vi "Capture Image.vi"(8 "Error In":errorcluster) -> (0 "Error Out":errorcluster)   [LabVIEW 2014]
uses:
  <vilib>/httpClient/LabVIEWHTTPClient.lvlib
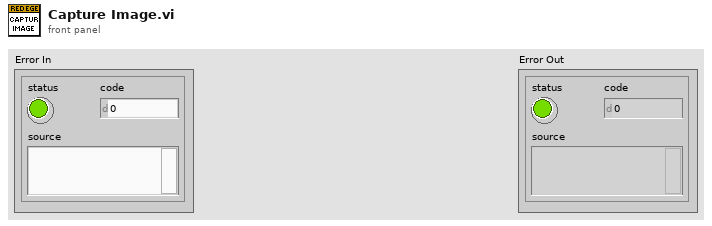
[diagram p1: front panel]
types:
  T1 = typedef "LabVIEWHTTPClient.lvlib/ClientHandle.ctl" = refnum<k1>
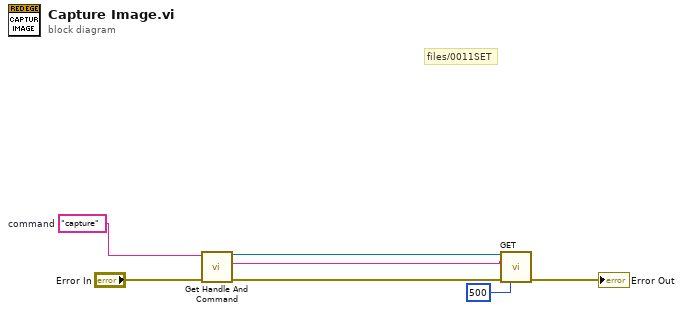
[diagram p0: block diagram]
diagram:
  w4 = "capture"  # command
  # "files/0011SET"
  n1 = call "Get Handle And Command.vi"("Error In"="Error In", "Command"=w4) -> ("Error Out"=w6:errorcluster, "Command URL"=w5:string, "RedEdge client handle out"=w7:T1)  [unwired: 6 in]
  n2 = call <vilib>:"GET.vi"("client handle"=w7, "url"=w5, "error in (no error)"=w6, "timeout (10000)"=500) -> ("error out"=→"Error Out":errorcluster)  [unwired: 8 in, 3 out]
